vi "前后侧IOT数据信息更新.vi"(8 "前/后侧":bool, 10 "IOT数据信息":T1, 11 "选项":T3) -> (1 "后侧IOT数据信息":T1, 3 "前侧IOT数据信息":T1)   [LabVIEW 2017]
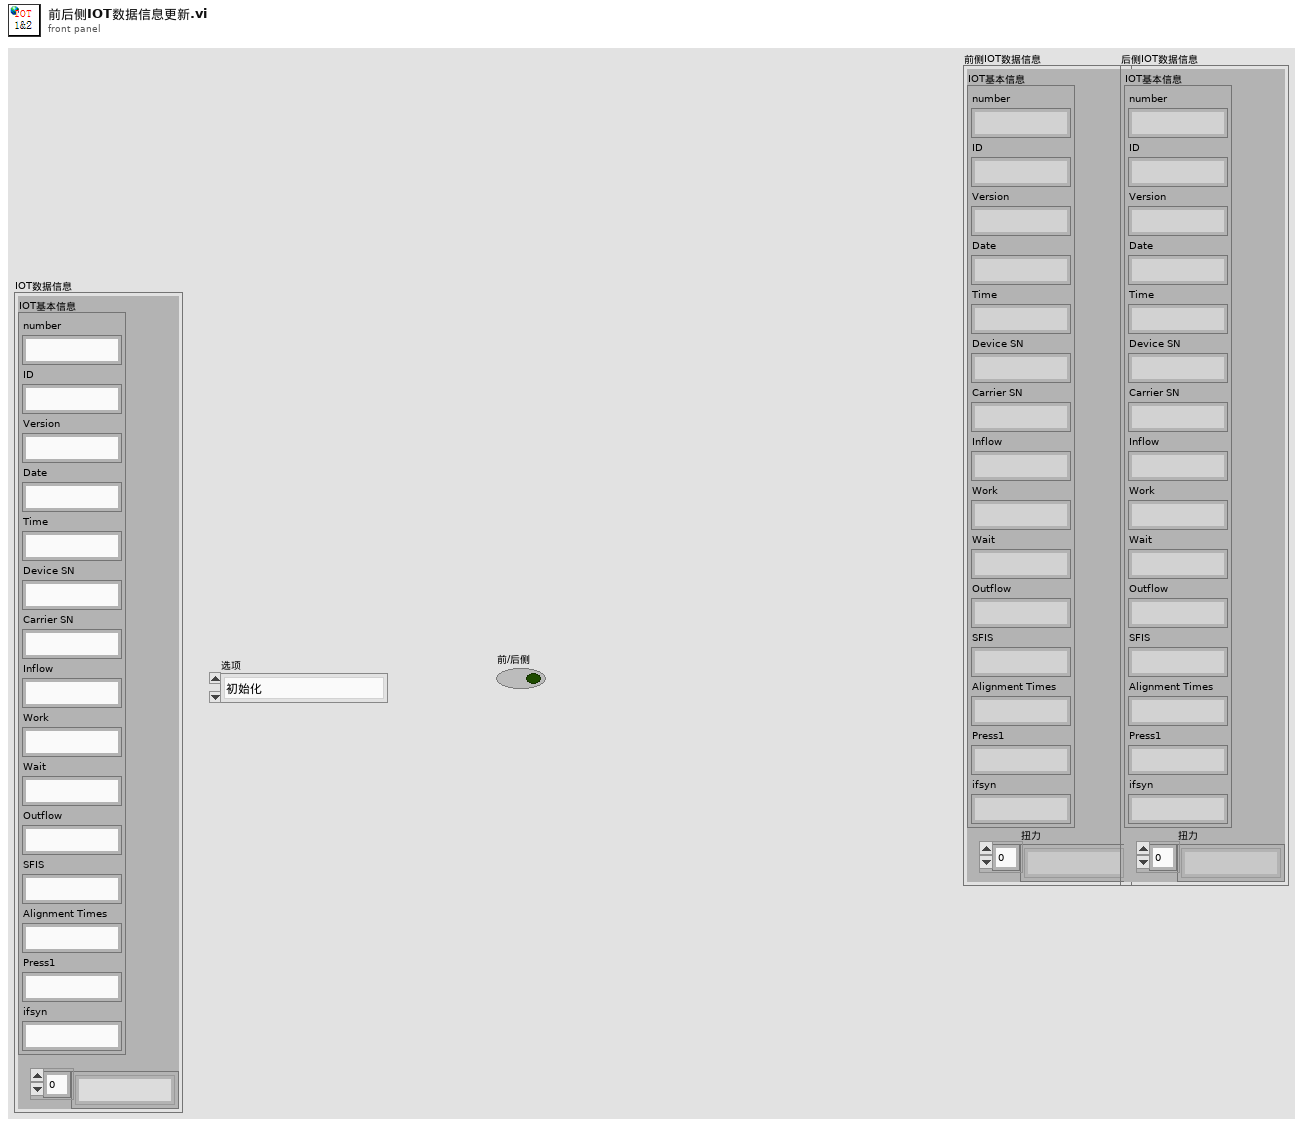
[diagram p1: front panel]
types:
  T1 = typedef "螺丝机IOT数据信息.ctl" = cluster{"IOT基本信息":T2, "扭力":string[]}
  T2 = typedef "IOT数据基本信息.ctl" = cluster{"number":string, "ID":string, "Version":string, "Date":string, "Time":string, "Device SN":string, "Carrier SN":string, "Inflow":string, "Work":string, "Wait":string, "Outflow":string, "SFIS":string, "Alignment Times":string, "Press1":string, "ifsyn":string}
  T3 = typedef "IOT数据更新选项.ctl" = enum16{"初始化", "更新数据", "获取寄存器", "前后站信息交互", "更新前站inflow&barcode"}
  T4 = typedef "提取参数项目.ctl" = enum16{"初始化", "基准拍照点提取", "物理距离信息提取", "锁附总表参数提取", "图纸锁附坐标提取", "更新图面offset", "图纸投影至机械", "提取数据"}
  T5 = typedef "参数集合.ctl" = cluster{"主&辅助定位孔拍照位置":T6, "物距提取信息":T8, "锁附总表参数":T11, "图面投影后检索结果":T16}
  T6 = typedef "主&辅助定位孔拍照位置.ctl" = cluster{"主定位孔拍照位置":T7, "辅助定位孔拍照位置":T7}
  T7 = typedef "定位孔拍照位置.ctl" = cluster{"动子位置":dbl, "供料轴位置":dbl, "Z轴位置":dbl}
  T8 = typedef "物距提取信息.ctl" = cluster{"物距":T9, "橡皮泥标记点":T7, "物距文档检索状态":T10, "标记拍照Z轴":dbl}
  T9 = typedef "物理距离.ctl" = cluster{"动子方向":dbl, "供料轴方向":dbl}
  T10 = typedef "总表检索状态.ctl" = enum16{"检索点位顺序超出范围", "检索OK"}
  T11 = typedef "锁附参数.ctl" = cluster{"锁附扭力":dbl, "锁附位置参数":T12, "锁附速度":T13, "锁附检测类参数":T14, "锁附点位编号":string, "总表检索状态":T10, "锁附总颗数":dbl, "起子编号":T15, "顺序编号":dbl, "组装孔？":bool, "扭力offset":dbl, "设定扭力":dbl, "锁附自救屏蔽？":bool}
  T12 = typedef "锁附位置参数.ctl" = cluster{"动子位置":dbl, "供料轴位置":dbl, "阶梯高度位置":dbl, "锁附深度":dbl}
  T13 = typedef "锁附速度.ctl" = cluster{"驱动速度":dbl, "加速度":dbl}
  T14 = typedef "锁附检测类参数.ctl" = cluster{"报警功能屏蔽？":bool, "锁附设定时间":dbl, "浮锁检测高度":dbl, "浮锁检测容差":dbl}
  T15 = typedef "起子编号.ctl" = enum16{"NA", "driver01", "driver02", "driver03", "driver04"}
  T16 = typedef "图面投影后检索结果.ctl" = cluster{"图纸投影后点位坐标":T9, "图面投影后文件检索状态":T10, "offset获取辅助集合":T17}
  T17 = typedef "offset获取辅助集合.ctl" = cluster{"offset获取半径spec":T18, "拍照高度":dbl, "曝光时间":dbl}
  T18 = typedef "上下限.ctl" = cluster{"上限":dbl, "下限":dbl}
  T19 = typedef "barcode结果显示.ctl" = cluster{"scanok?":bool, "barcode":string, "Time":dbl, "锁附OK?":bool, "SN":string}
  T20 = cluster{"%Y_%m_%d_%H_%M_%S%3u":string, "%Y_%m_%d":string, "%H_%M_%S%3u":string}
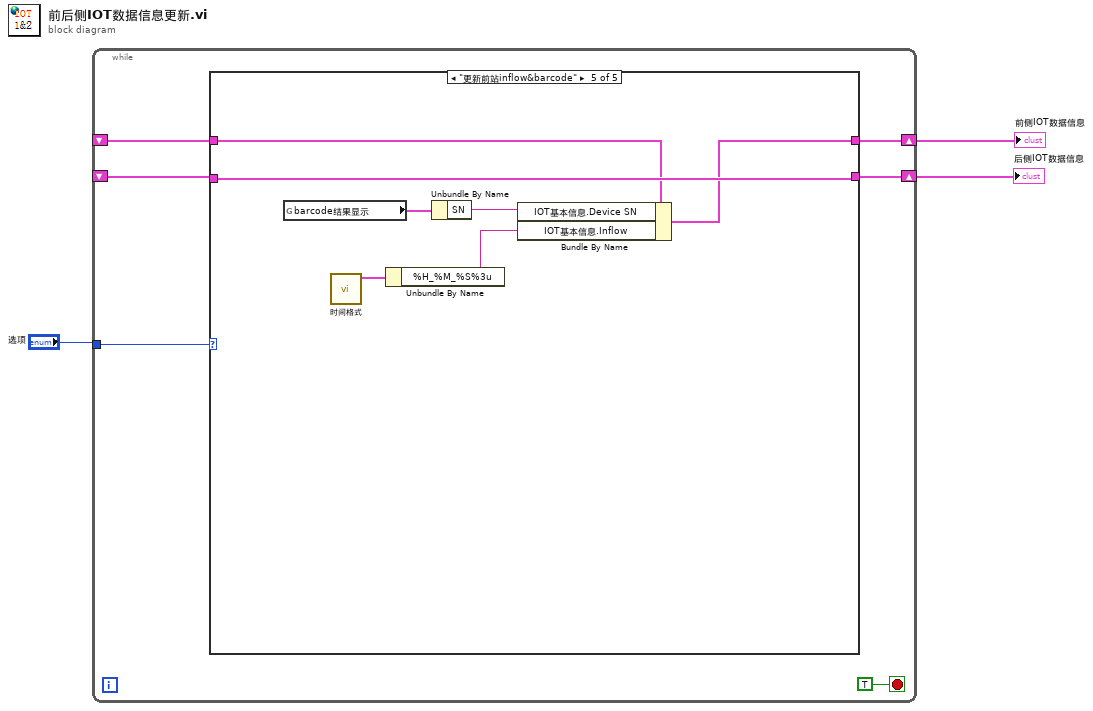
[diagram p0: block diagram]
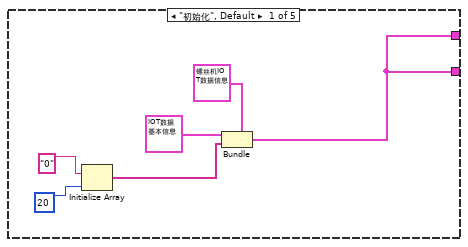
[diagram p2: hidden frame]
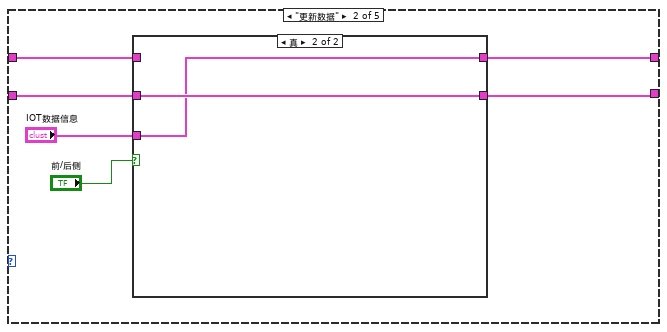
[diagram p3: hidden frame]
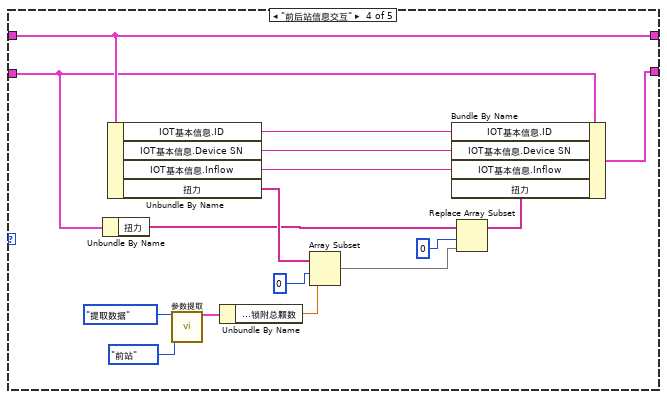
[diagram p6: hidden frame]
diagram:
  n1 = while {
    tunnel: "选项" -> [w8]
    shift-right: [w6] -> w2
    shift-left: _ -> [w5]
    shift-right: [w7] -> w1
    shift-left: _ -> [w4]
    stop <- TRUE stop-if-true
    n2 = case shown="\"更新前站inflow&barcode\"" w8 {
      tunnel: [w12 w16 w27 w43 w48] -> w6
      tunnel: [w12 w18 w26 w40 w50] -> w7
      tunnel: w5 -> [_ w20 w27 w43 w49]
      tunnel: w4 -> [_ w19 w26 w37 w50]
      frame "初始化", Default {
        n3 = Initialize Array("0", 20 ("维数大小")) -> (w13:string[])
        n4 = Bundle(cluster=T1 {"IOT基本信息"={"number"="", "ID"="", "Version"="", "Date"="", "Time"="", "Device SN"="", "Carrier SN"="", "Inflow"="", "Work"="", "Wait"="", "Outflow"="", "SFIS"="", "Alignment Times"="", "Press1"="", "ifsyn"=""}, "扭力"=[]} ("IOT数据信息 2"), "IOT基本信息"=T2 {"number"="", "ID"="", "Version"="", "Date"="", "Time"="", "Device SN"="", "Carrier SN"="", "Inflow"="", "Work"="", "Wait"="", "Outflow"="", "SFIS"="", "Alignment Times"="", "Press1"="", "ifsyn"="N"}, "扭力"=w13) -> (w12:T1)
      }
      frame "更新数据" {
        n5 = case shown="真" "前/后侧" {
          tunnel: [w23 w24] -> w16
          tunnel: w20 -> [w23 _]
          tunnel: w19 -> [_ w25]
          tunnel: [w22 w25] -> w18
          tunnel: "IOT数据信息" -> [w22 w24]
          frame False {
          }
          frame True {
          }
        }
      }
      frame "获取寄存器" {
      }
      frame "前后站信息交互" {
        n6 = Unbundle By Name(w37) -> ("扭力"=w36:string[])
        n7 = Unbundle By Name(w43) -> ("IOT基本信息.ID"=w28:string, "IOT基本信息.Device SN"=w42:string, "IOT基本信息.Inflow"=w41:string, "扭力"=w39:string[])
        n8 = call "参数提取.vi"("提取参数项目"=提取参数项目."提取数据", "前/后站"=enum16{"前站", "后站"}."前站") -> ("参数集合out"=w30:T5)  [unwired: 10 in, 3 out]
        n9 = Unbundle By Name(w30) -> ("锁附总表参数.锁附总颗数"=w29:dbl)
        n10 = Array Subset(array=w39, index=0 ("索引"), length=w29) -> (w35:string[])
        n11 = Replace Array Subset(array=w36, new element=w35, index=0 ("索引")) -> (w33:string[])
        n12 = Bundle By Name(cluster=w37, "IOT基本信息.ID"=w28, "IOT基本信息.Device SN"=w42, "IOT基本信息.Inflow"=w41, "扭力"=w33) -> (w40:T1)
      }
      frame "更新前站inflow&barcode" {
        n13 = global read "读码器全局.vi" "barcode结果显示"() -> (w45:T19)
        n14 = call "时间格式.vi"() -> ("时间格式"=w47:T20)  [unwired: 11 in]
        n15 = Unbundle By Name(w47) -> ("%H_%M_%S%3u"=w46:string)
        n16 = Unbundle By Name(w45) -> ("SN"=w44:string)
        n17 = Bundle By Name(cluster=w49, "IOT基本信息.Device SN"=w44, "IOT基本信息.Inflow"=w46) -> (w48:T1)
      }
    }
  }
  "前侧IOT数据信息" <- w2
  "后侧IOT数据信息" <- w1
